vi "SaveToFile.vi"(0 "file path (dialog if empty)":path, 1 "MagX_A":refnum<vi>, 3 "MagY_A":refnum<vi>, 4 "MagZ_A":refnum<vi>, 5 "Y_Accel g":ext format="%#_4g", 6 "X_Accel g":ext format="%#_4g", 9 "Z_Accel g":ext format="%#_4g", 10 "Z_Mag":ext format="%#_4g", 11 "X_Mag":ext format="%#_4g", 12 "Y_Mag":ext format="%#_4g", 13 "BIT_T":bool, 14 "M[mgauss]":ext, 15 "BIT":u16) -> ()   [LabVIEW 2017]
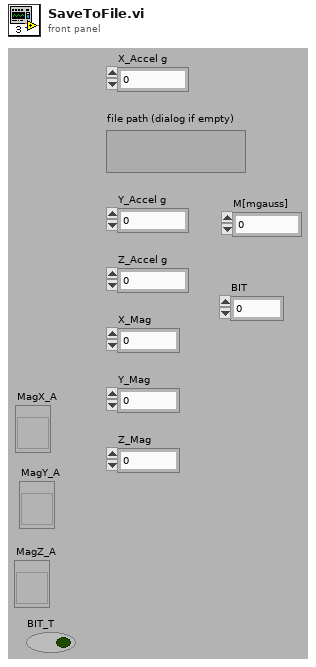
[diagram p1: front panel]
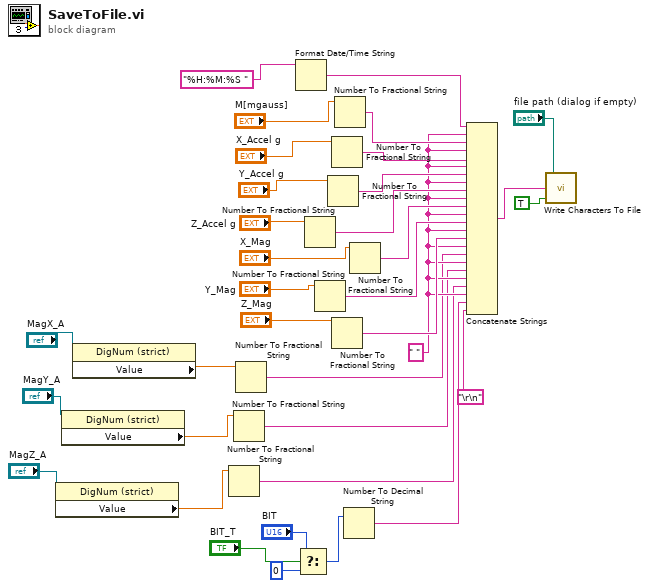
[diagram p0: block diagram]
diagram:
  w11 = " "
  n1 = property class="DigNum (strict)"(reference="MagZ_A") -> ("Value"=w8:dbl)  [unwired: 1 in, 2 out]
  n2 = property class="DigNum (strict)"(reference="MagY_A") -> ("Value"=w9:dbl)  [unwired: 1 in, 2 out]
  n3 = property class="DigNum (strict)"(reference="MagX_A") -> ("Value"=w10:dbl)  [unwired: 1 in, 2 out]
  n4 = Number To Fractional String(number=w8) -> (F-format string=w5:string)  [unwired: 3 in]
  n5 = Number To Fractional String(number=w9) -> (F-format string=w6:string)  [unwired: 3 in]
  n6 = Number To Fractional String(number=w10) -> (F-format string=w7:string)  [unwired: 3 in]
  n7 = Format Date/Time String(time format string (%c)="%H:%M:%S ") -> (date/time string=w16:string)  [unwired: 2 in]
  n8 = Select(t="BIT", s="BIT_T", f=u16 0) -> (s? t:f=w3:u16)
  n9 = Number To Fractional String(number="Z_Accel g") -> (F-format string=w28:string)  [unwired: 3 in]
  n10 = Number To Fractional String(number="Y_Mag") -> (F-format string=w30:string)  [unwired: 3 in]
  n11 = Number To Fractional String(number="Y_Accel g") -> (F-format string=w27:string)  [unwired: 3 in]
  n12 = Number To Fractional String(number="X_Accel g") -> (F-format string=w26:string)  [unwired: 3 in]
  n13 = Number To Fractional String(number="Z_Mag") -> (F-format string=w31:string)  [unwired: 3 in]
  n14 = Number To Fractional String(number="M[mgauss]") -> (F-format string=w15:string)  [unwired: 3 in]
  n15 = Number To Decimal String(number=w3) -> (decimal integer string=w18:string)  [unwired: 1 in]
  n16 = Number To Fractional String(number="X_Mag") -> (F-format string=w29:string)  [unwired: 3 in]
  n17 = Concatenate Strings(w16, w11, w15, w11, w26, w11, w27, w11, w28, w11, w29, w11, w30, w11, w31, w11, w7, w11, w6, w11, w5, w11, w18, "\r\n") -> (w33:string)
  n18 = call <vilib>:"Write Characters To File.vi"("append to file? (new file:F)"=TRUE, "character string"=w33, "file path (dialog if empty)"="file path (dialog if empty)") -> ()  [unwired: 2 in, 1 out]
